vi "Pfeiffer Vacuum Date-Time of listed Errors.vi"(8 "error in (no error)":errorcluster, 9 "Position :":u16=1 min=1 max=10 step=1, 10 "Adress of unit":u16=1 min=1 max=999 step=1, 11 "VISA session in":refnum<visa-resource-name>) -> (0 "error out":errorcluster, 3 "response (data)":string)   [LabVIEW 2018]
doc: "This VI is an example of how to use the Pfeiffer Vacuum subVIs programmatically. This VI first initializes the instrument, takes measurements, then closes the instrument."
uses:
  <instrlib>/Pfeiffer Vacuum/Pfeiffer Vacuum.lvlib
panel:
  # "Read time / date of listed\nerror storage at"
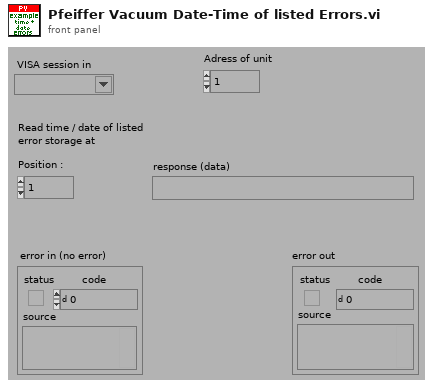
[diagram p1: front panel]
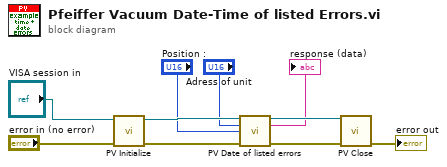
[diagram p0: block diagram]
diagram:
  n1 = call <instrlib>:"PV Initialize.vi"("error in (no error)"="error in (no error)", "VISA session in"="VISA session in") -> ("error out"=w10:errorcluster, "VISA session out"=w8:refnum<visa-resource-name>)  [unwired: 8 in]
  n2 = call <instrlib>:"PV Date of listed errors.vi"("VISA session"=w8, "Adress of unit"="Adress of unit", "Position :"="Position :", "error in (no error)"=w10) -> ("dup VISA session"=w7:refnum<visa-resource-name>, "response (data)"=→"response (data)":string, "error out"=w9:errorcluster)  [unwired: 9 in]
  n3 = call <instrlib>:"PV Close.vi"("VISA session"=w7, "error in (no error)"=w9) -> ("error out"=→"error out":errorcluster)  [unwired: 13 in]
